vi "AdquisicioDadesUSB.vi"(8 "Stop":refnum<vi>, 11 "user event out":refnum<user-event>) -> ()   [LabVIEW 2017]
uses:
  <vilib>/DAQmx/read.llb/DAQmx Read (Digital 1D Bool NChan 1Samp 1Line).vi
  <vilib>/DAQmx/read.llb/DAQmx Read (Analog 1D DBL 1Chan NSamp).vi
  <vilib>/DAQmx/miscellaneous.llb/DAQmx Fill In Error Info.vi
  <resource>/objmgr/daqmx.rc
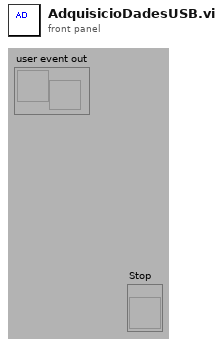
[diagram p1: front panel]
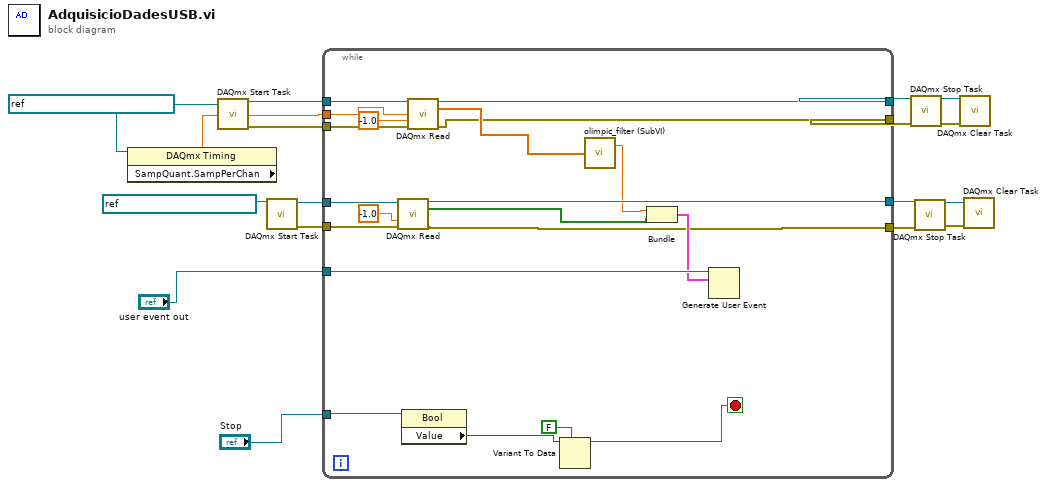
[diagram p0: block diagram]
diagram:
  w11 = refnum<k21> "TallGuants_USBDAnalogIn" ("task/channels in")
  n1 = property class="DAQmx Timing"(reference=w11) -> ("SampQuant.SampPerChan"=w17:dbl)  [unwired: 1 in, 2 out]
  n2 = call <vilib>:"DAQmx Start Task.vi"("task/channels in"=w11) -> ("task out"=w15:refnum<k21>, "error out"=w14:errorcluster)  [unwired: 13 in]
  n3 = call <vilib>:"DAQmx Start Task.vi"("task/channels in"=refnum<k21> "TallGuants_USBDigitalIn") -> ("task out"=w9:refnum<k21>, "error out"=w1:errorcluster)  [unwired: 13 in]
  n4 = while {
    tunnel: w15 -> [w29]
    tunnel: w17 -> [w31]
    tunnel: [w30] -> w16
    tunnel: w14 -> [w37]
    tunnel: "Stop" -> [w36]
    tunnel: [w19] -> w12
    tunnel: w9 -> [w27]
    tunnel: [w26] -> w8
    tunnel: [w20] -> w7
    tunnel: "user event out" -> [w25]
    tunnel: w1 -> [w21]
    stop <- w33 stop-if-true
    n5 = call-poly <vilib>:"DAQmx Read.vi"("task/channels in"=w27, "timeout"=-1.0, "error in"=w21) -> ("task out"=w26:refnum<k21>, "data"=w23:bool[], "error out"=w20:errorcluster)  [unwired: 10 in]
    n6 = property class="Bool"(reference=w36) -> ("Value"=w35:variant)  [unwired: 1 in, 2 out]
    n7 = call-poly <vilib>:"DAQmx Read.vi"("task/channels in"=w29, "number of samples per channel"=w31, "timeout"=-1.0, "error in"=w37) -> ("task out"=w30:refnum<k21>, "data"=w28:dbl[], "error out"=w19:errorcluster)  [unwired: 9 in]
    n8 = Variant To Data(type=FALSE, Variant=w35) -> (data=w33:bool)  [unwired: 1 in, 1 out]
    n9 = call "olimpic_filter (SubVI).vi"("array"=w28) -> ("olimpic_filter"=w24:dbl)  [unwired: 1 out]
    n10 = Bundle("olimpic_filter"=w24, "data"=w23) -> (w22:cluster{"olimpic_filter":dbl, "data":bool[]})  [unwired: 1 in]
    n11 = Generate User Event(user event=w25, event data cluster=w22) -> ()  [unwired: 2 in, 2 out]
  }
  n12 = call <vilib>:"DAQmx Stop Task.vi"("task/channels in"=w16, "error in"=w12) -> ("task out"=w5:refnum<k21>, "error out"=w4:errorcluster)  [unwired: 12 in]
  n13 = call <vilib>:"DAQmx Stop Task.vi"("task/channels in"=w8, "error in"=w7) -> ("task out"=w3:refnum<k21>, "error out"=w2:errorcluster)  [unwired: 12 in]
  n14 = call <vilib>:"DAQmx Clear Task.vi"("task in"=w5, "error in"=w4) -> ()  [unwired: 13 in, 1 out]
  n15 = call <vilib>:"DAQmx Clear Task.vi"("task in"=w3, "error in"=w2) -> ()  [unwired: 13 in, 1 out]
